vi "Agilent_33220A_FuncGen_TCP_3.vi"() -> ()   [LabVIEW 2019, in "Models of External Instruments.lvlib"]
uses:
  Models of External Instruments.lvlib
panel:
  out "remote port":u16
  out "remote address":string
  out "data out":string
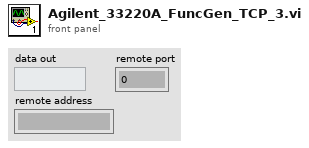
[diagram p1: front panel]
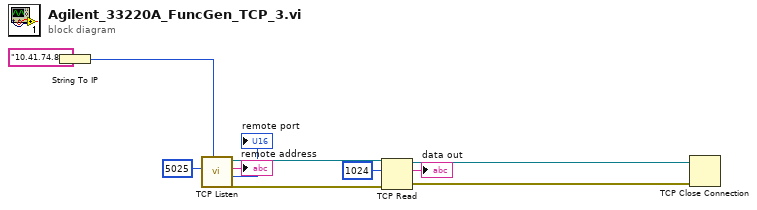
[diagram p0: block diagram]
diagram:
  n1 = String To IP(1:"10.41.74.80") -> (0:w3:u32)
  n2 = call <vilib>:"TCP Listen.vi"("net address"=w3, "port"=u16 5025) -> ("error out"=w10:errorcluster, "remote port"=→"remote port":u16, "remote address"=→"remote address":string, "connection ID"=w11:refnum<k5>)  [unwired: 5 in, 1 out]
  n3 = TCP Read(connection ID=w11, bytes to read=1024, error in (no error)=w10) -> (connection ID out=w9:refnum<k5>, data out=→"data out":string, error out=w8:errorcluster)  [unwired: 2 in]
  n4 = TCP Close Connection(connection ID=w9, error in (no error)=w8) -> ()  [unwired: 1 in, 2 out]
